vi "Disable.vi"(10 "error in":errorcluster) -> (2 "error out":errorcluster)   [LabVIEW 2022 SP3]
uses:
  Newport.XPS.CommandInterface
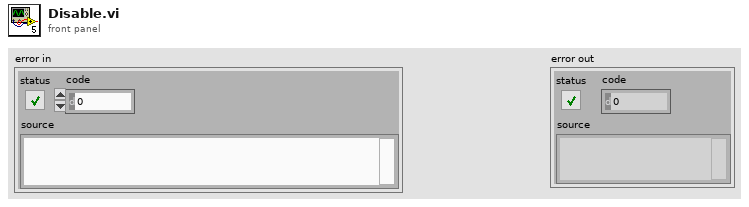
[diagram p1: front panel]
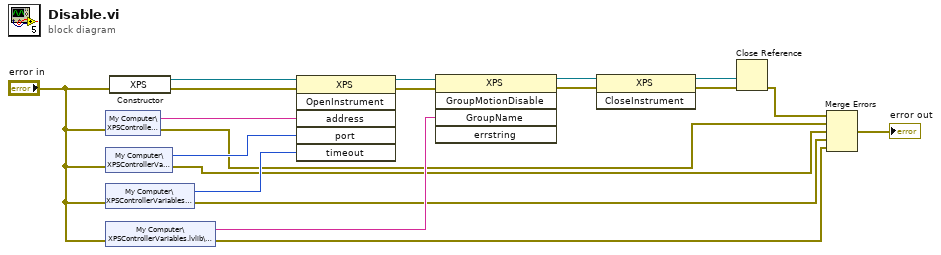
[diagram p0: block diagram]
diagram:
  n1 = shared-variable "My Computer\\XPSControllerVariables.lvlib\\IP"(error in="error in") -> (w15:string, error out=w9:errorcluster)
  n2 = shared-variable "My Computer\\XPSControllerVariables.lvlib\\Port"(error in="error in") -> (w13:i16, error out=w8:errorcluster)
  n3 = shared-variable "My Computer\\XPSControllerVariables.lvlib\\Timeout"(error in="error in") -> (w12:i16, error out=w7:errorcluster)
  n4 = shared-variable "My Computer\\XPSControllerVariables.lvlib\\GroupName"(error in="error in") -> (w11:string, error out=w6:errorcluster)
  n5 = constructor class="XPS"(error in="error in") -> (reference out=w18:refnum<k24>, error out=w19:errorcluster)  [unwired: 2 in, 1 out]
  n6 = invoke class="XPS" method="OpenInstrument"(reference=w18, error in=w19, "address"=w15, "port"=w13, "timeout"=w12) -> (reference out=w4:refnum<k24>, error out=w3:errorcluster)  [unwired: 1 in, 4 out]
  n7 = invoke class="XPS" method="GroupMotionDisable"(reference=w4, error in=w3, "GroupName"=w11) -> (reference out=w2:refnum<k24>, error out=w1:errorcluster)  [unwired: 2 in, 3 out]
  n8 = invoke class="XPS" method="CloseInstrument"(reference=w2, error in=w1) -> (reference out=w17:refnum<k24>, error out=w16:errorcluster)  [unwired: 1 in, 1 out]
  n9 = Close Reference(reference=w17, error in (no error)=w16) -> (error out=w10:errorcluster)
  n10 = Merge Errors(w10, w9, w8, w7, w6) -> (→"error out":errorcluster)
